vi "OpenFPGARef.vi"(8 "error in":errorcluster, 11 "FPGASession in":refnum<class "FPGASession.lvclass">) -> (0 "error out":errorcluster, 3 "FPGASession out":refnum<class "FPGASession.lvclass">)   [LabVIEW 2013, in "FPGASession.lvclass"]
uses:
  FPGASession.lvclass
  <vilib>/rvi/interface/nirviOpenFPGA/nirviOpenFPGA.xnode
  RT/FPGASession/FPGARef.ctl
  FPGATargetClass/FPGATarget.lvclass
  FPGA Bitfiles/HWSWTriggerBox_FPGATarget2_TriggerBox_1zhzIx5zPP8.lvbitx
  FPGAMain.vi
  <vilib>/FPGAPlugInAG/sbRIO-9636/niLvFpga_Open_sbRIO-9636.vi
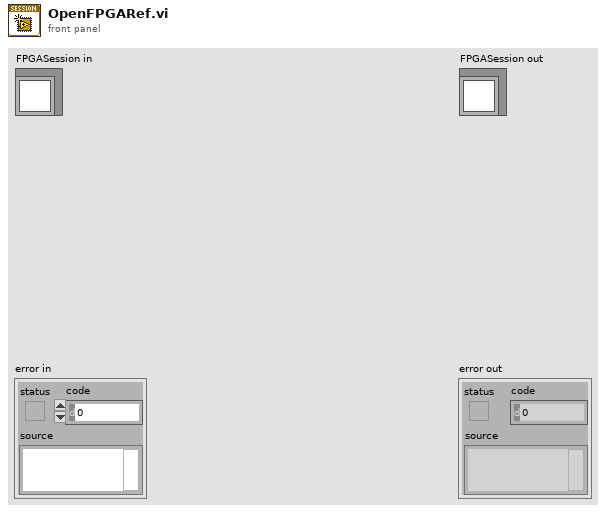
[diagram p1: front panel]
types:
  T1 = typedef "nirio_resource_hc.ctl" = tag
  T2 = typedef "FPGASession.lvclass/FPGARef.ctl" = refnum<k20>
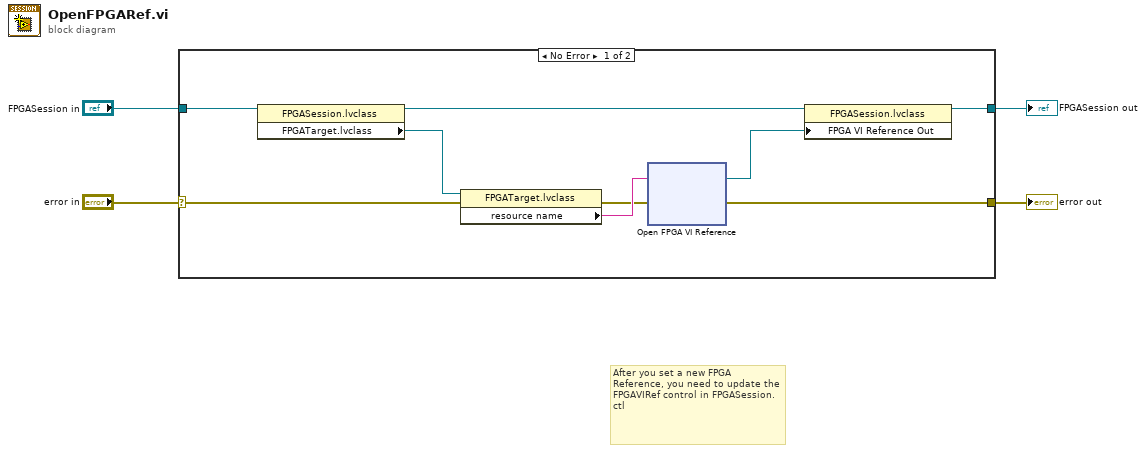
[diagram p0: block diagram]
diagram:
  # "After you set a new FPGA Reference, you need to update the FPGAVIRef control in FPGASession.ctl"
  n1 = case shown="No Error" "error in" {
    selector: "error in" -> [w12 w15]
    tunnel: [w10 w15] -> w3
    tunnel: [w9 w14] -> w1
    tunnel: "FPGASession in" -> [w7 w14]
    frame No Error {
      n2 = property class="FPGASession.lvclass"(reference=w7) -> (reference out=w6:refnum<class "FPGASession.lvclass">, "FPGATarget.lvclass"=w5:refnum<class "FPGATarget.lvclass">)  [unwired: 1 in, 1 out]
      n3 = property class="FPGATarget.lvclass"(reference=w5, error in=w12) -> (error out=w11:errorcluster, "resource name"=w13:T1)  [unwired: 1 out]
      n4 = xnode "Open FPGA VI Reference"("error in"=w11, "resource name"=w13) -> ("FPGA VI Reference Out"=w8:T2, "error out"=w10:errorcluster)
      n5 = property class="FPGASession.lvclass"(reference=w6, "FPGA VI Reference Out"=w8) -> (reference out=w9:refnum<class "FPGASession.lvclass">)  [unwired: 1 in, 1 out]
    }
    frame Error {
    }
  }
  "error out" <- w3
  "FPGASession out" <- w1
